vi "ProcessState-WaitOnStoppped.vi"(2 "PROCESS":string, 9 "error in (no error)":errorcluster) -> (6 "error out":errorcluster)   [LabVIEW 2009]
uses:
  ProcessState.ctl
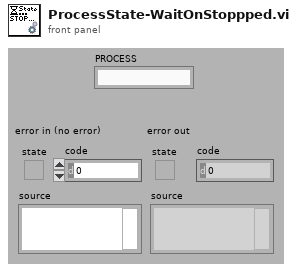
[diagram p1: front panel]
types:
  T1 = typedef "ProcessState.ctl" = enum16{"STARTING", "RUNNING", "STOPPING", "STOPPPED"}
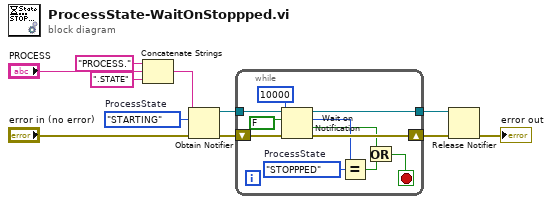
[diagram p0: block diagram]
diagram:
  w9 = ProcessState."STARTING"  # ProcessState
  n1 = Concatenate Strings("PROCESS." ("chaîne"), "PROCESS", ".STATE" ("chaîne")) -> (w11:string)
  n2 = Obtain Notifier(name (unnamed)=w11, notification data type=w9, error in (no error)="error in (no error)") -> (notifier out=w5:refnum<notifier>, error out=w6:errorcluster)  [unwired: 1 in, 1 out]
  n3 = while {
    tunnel: w5 -> [w21]
    tunnel: [w16] -> w3
    shift-right: [w20] -> w4
    shift-left: w6 -> [w22]
    stop <- w12 stop-if-true
    w17 = ProcessState."STOPPPED"  # ProcessState
    n4 = Wait on Notification(notifier=w21, ignore previous (F)=FALSE ("ignorer précédent (F)"), timeout in ms (-1)=10000 ("timeout en ms (-1)"), error in (no error)=w22) -> (notifier out=w16:refnum<notifier>, notification=w18:T1, timed out?=w13:bool, error out=w20:errorcluster)
    n5 = Equal?(x=w18, y=w17) -> (x = y?=w14:bool)
    n6 = Or(x=w13, y=w14) -> (x .or. y?=w12:bool)
  }
  n7 = Release Notifier(notifier=w3, error in (no error)=w4) -> (error out=→"error out":errorcluster)  [unwired: 3 out]
